vi "HealthCheckBigHPPT (1).vi"(1 "Numeric":dbl) -> (0 "Boolean":bool)   [LabVIEW 2017]
uses:
  NominalRangeGLOBAL.vi
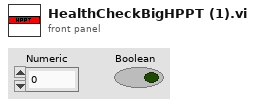
[diagram p1: front panel]
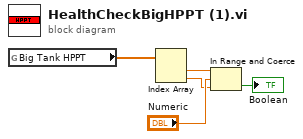
[diagram p0: block diagram]
diagram:
  n1 = global read "NominalRangeGLOBAL.vi" "Big Tank HPPT"() -> (w3:dbl[])
  n2 = Index Array(array=w3) -> (element #1=w2:dbl, element #2=w1:dbl)  [unwired: 2 in]
  n3 = In Range and Coerce(upper limit=w2, x="Numeric", lower limit=w1) -> (In Range?=→"Boolean":bool)  [unwired: 1 out]
